vi "Model.vi"(8 "error in (no error)":errorcluster, 10 "Input onfiguration":T1={"Input File Path"=path "", "from scan..."=0, "...to scan"=0, "Resistance in series"=0.0, "Correct conductance "=FALSE, "Model parameters gap 1"={"Delta 1"=0.0, "Delta 2"=0.0, "Gama"=0.0, "Z"=0.0, "P"=0.0, "T"=0.0, "Integration range"=0.0, "Resolution"=0.0}, "Scale"=0.0, "Offset"=0.0, "Append channels"=[], "Model parameters gap 2"={"Delta 1"=0.0, "Delta 2"=0.0, "Gama"=0.0, "Z"=0.0, "P"=0.0, "T"=0.0, "Integration range"=0.0, "Resolution"=0.0}, "Gap 2 weight"=0.0, "Gnormal"=0.0, "Channels"=["V", "I", "dIdV"], "Preserve model history"=FALSE} {"Gnormal" step=0.0001 format="%#_6p"; "Model parameters gap 2"."Delta 1" step=0.001 format="%#_6peV"; "Model parameters gap 2"."Resolution" format="%#_6peV"; "Model parameters gap 2"."Integration range" format="%#_6peV"; "Model parameters gap 2"."T" format="%#_6pK"; "Model parameters gap 2"."Delta 2" step=0.001 format="%#_6peV"; "Model parameters gap 2"."Gama" step=0.001 format="%#_6peV"; "Offset" scale=0.0..0.1; "Scale" scale=0.0..0.03; "Model parameters gap 1"."Delta 1" step=0.001 format="%#_6peV"; "Model parameters gap 1"."Resolution" format="%#_6peV"; "Model parameters gap 1"."Integration range" format="%#_6peV"; "Model parameters gap 1"."T" format="%#_6pK"; "Model parameters gap 1"."Delta 2" step=0.001 format="%#_6peV"; "Model parameters gap 1"."Gama" step=0.001 format="%#_6peV"; "Resistance in series" scale=0.0..80.0}, 11 "dIdV State in":refnum<class "Point Contact Model.lvclass">) -> (0 "error out":errorcluster, 3 "dIdV State out":refnum<class "Point Contact Model.lvclass">)   [LabVIEW 2021, in "Point Contact Model.lvclass"]
uses:
  Point Contact Model.lvclass
  Controls/PCS Config.ctl
  Parameters.ctl
  Point Contact Model.lvclass/Point Contact Model.ctl
panel:
  # "V"
  # "I"
  # "dIdV"
  # "<="
  # "<="
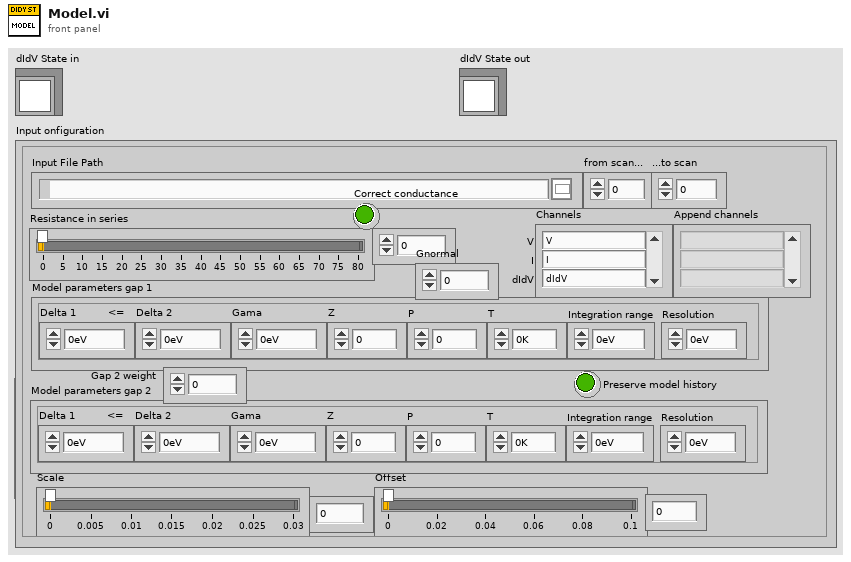
[diagram p1: front panel]
types:
  T1 = typedef "PCS Config.ctl" = cluster{"Input File Path":path, "from scan...":i32, "...to scan":i32, "Resistance in series":dbl, "Correct conductance ":bool, "Model parameters gap 1":T2, "Scale":dbl, "Offset":dbl, "Append channels":string[], "Model parameters gap 2":T2, "Gap 2 weight":dbl, "Gnormal":dbl, "Channels":string[], "Preserve model history":bool}
  T2 = typedef "Parameters.ctl" = cluster{"Delta 1":dbl, "Delta 2":dbl, "Gama":dbl, "Z":dbl, "P":dbl, "T":dbl, "Integration range":dbl, "Resolution":dbl}
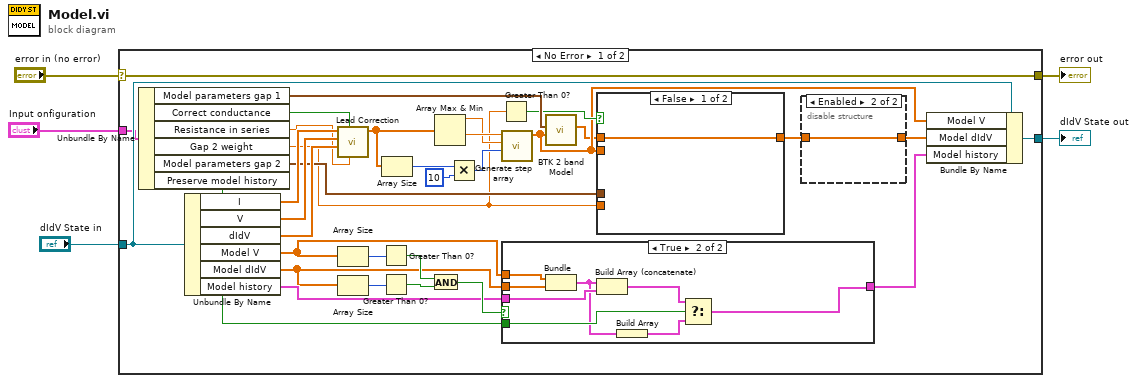
[diagram p0: block diagram]
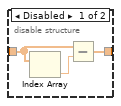
[diagram p3: hidden frame]
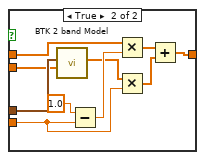
[diagram p4: hidden frame]
diagram:
  n1 = case shown="No Error" "error in (no error)" {
    selector: "error in (no error)" -> [w38 w64]
    tunnel: [w38 w64] -> w4
    tunnel: [w24 w63] -> w2
    tunnel: "dIdV State in" -> [w37 w63]
    tunnel: "Input onfiguration" -> [w33 _]
    frame No Error {
      n2 = Unbundle By Name(w33) -> ("Model parameters gap 1"=w30:T2, "Correct conductance"=w31:bool, "Resistance in series"=w32:dbl, "Gap 2 weight"=w17:dbl, "Model parameters gap 2"=w20:T2, "Preserve model history"=w6:bool)
      n3 = Unbundle By Name(w37) -> ("I"=w36:dbl[], "V"=w35:dbl[], "dIdV"=w34:dbl[], "Model V"=w9:dbl[], "Model dIdV"=w8:dbl[], "Model history"=w10:cluster{"Model V":dbl[], "Model dIdV":dbl[]}[])
      n4 = call "Lead Correction.vi"("Resistance in series"=w32, "Correct conductance"=w31, "dIdV"=w34, "V"=w35, "I"=w36) -> ("V out"=w23:dbl[])  [unwired: 3 in, 3 out]
      n5 = Array Size(array=w9) -> (size(s)=w15:i32)
      n6 = Array Size(array=w8) -> (size(s)=w14:i32)
      n7 = Greater Than 0?(x=w15) -> (x > 0?=w13:bool)
      n8 = Greater Than 0?(x=w14) -> (x > 0?=w12:bool)
      n9 = Array Size(array=w23) -> (size(s)=w27:i32)
      n10 = And(x=w13, y=w12) -> (x .and. y?=w11:bool)
      n11 = Array Max & Min(array=w23) -> (max value=w25:dbl, min value=w26:dbl)  [unwired: 2 out]
      n12 = Multiply(x=w27, y=10) -> (x*y=w28:i32)
      n13 = Greater Than 0?(x=w17) -> (x > 0?=w21:bool)
      n14 = call "Generate step array.vi"("Number of steps"=w28, "End"=w25, "Start"=w26) -> ("Steps"=w19:dbl[])  [unwired: 8 in]
      n15 = case shown="True" w11 {
        tunnel: w10 -> [w39 w47]
        tunnel: w9 -> [_ w46]
        tunnel: w8 -> [_ w45]
        tunnel: [w39 w40] -> w7
        tunnel: w6 -> [_ w44]
        frame False {
        }
        frame True {
          n16 = Bundle("Model V"=w46, "Model dIdV"=w45) -> (w43:cluster{"Model V":dbl[], "Model dIdV":dbl[]})  [unwired: 1 in]
          n17 = Build Array (concatenate)(w43, w47) -> (w41:cluster{"Model V":dbl[], "Model dIdV":dbl[]}[])
          n18 = Build Array(w43) -> (w42:cluster{"Model V":dbl[], "Model dIdV":dbl[]}[])
          n19 = Select(t=w41, s=w44, f=w42) -> (s? t:f=w40:cluster{"Model V":dbl[], "Model dIdV":dbl[]}[])
        }
      }
      n20 = call "BTK 2 band Model.vi"("V"=w19, "Parameters"=w30) -> ("Conductivity"=w18:dbl[])  [unwired: 9 in]
      n21 = case shown="False" w21 {
        tunnel: w20 -> [_ w62]
        tunnel: w19 -> [_ w61]
        tunnel: w18 -> [w52 w60]
        tunnel: w17 -> [_ w56]
        tunnel: [w52 w53] -> w16
        frame False {
        }
        frame True {
          n22 = call "BTK 2 band Model.vi"("V"=w61, "Parameters"=w62) -> ("Conductivity"=w57:dbl[])  [unwired: 9 in]
          n23 = Subtract(x=1.0, y=w56) -> (x-y=w58:dbl)
          n24 = Multiply(x=w60, y=w58) -> (x*y=w55:dbl[])
          n25 = Multiply(x=w57, y=w56) -> (x*y=w54:dbl[])
          n26 = Add(x=w55, y=w54) -> (x+y=w53:dbl[])
        }
      }
      n27 = disable-structure shown="Enabled" {
        disable-tunnel: [w49 w51] -> w22
        disable-tunnel: w16 -> [w48 w51]
        frame Disabled {
          n28 = Index Array(array=w48) -> (element=w50:dbl)  [unwired: 1 in]
          n29 = Subtract(x=w48, y=w50) -> (x-y=w49:dbl[])
        }
        frame Enabled {
        }
      }
      n30 = Bundle By Name(cluster=w37, "Model V"=w19, "Model dIdV"=w22, "Model history"=w7) -> (w24:refnum<class "Point Contact Model.lvclass">)
    }
    frame Error {
    }
  }
  "error out" <- w4
  "dIdV State out" <- w2
